vi "Get Shooter Queue.vi"(8 "error in (no error)":errorcluster) -> (0 "error out":errorcluster, 3 "Queue out":refnum<queue>)   [LabVIEW 2016]
uses:
  Shooterqueue.ctl
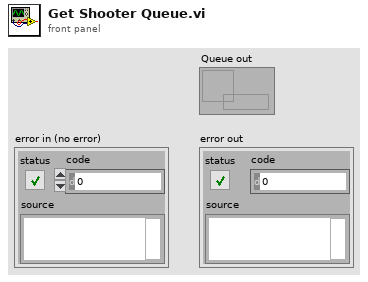
[diagram p1: front panel]
types:
  T1 = typedef "Shooterqueue.ctl" = cluster{"msg":string, "value":dbl}
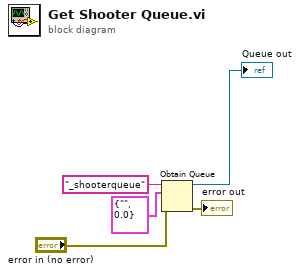
[diagram p0: block diagram]
diagram:
  n1 = Obtain Queue(name (unnamed)="_shooterqueue", element data type=T1 {"msg"="", "value"=0.0}, error in (no error)="error in (no error)") -> (queue out=→"Queue out":refnum<queue>, error out=→"error out":errorcluster)  [unwired: 2 in, 1 out]
